vi "SetTrigger.vi"(8 "error in (no error)":errorcluster, 10 "Settings.Trigger":T1, 11 "PCO in":refnum<class "PCO_Camera.lvclass">) -> (0 "error out":errorcluster, 2 "Settings.Trigger  out":T1, 3 "PCO out":refnum<class "PCO_Camera.lvclass">)   [LabVIEW 2020, in "PCO_Camera.lvclass"]
uses:
  PCO_Camera.lvclass
  OnOffTypeDef.ctl
  PCO_Camera.lvclass/PCO_Camera.ctl
  Camera.lvclass
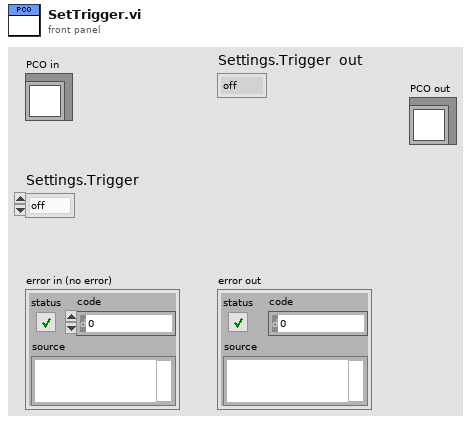
[diagram p1: front panel]
types:
  T1 = typedef "OnOffTypeDef.ctl" = enum16{"off", "on"}
  T2 = enum16{"sequence", "sequence non blocking", "ring buffer", "fifo", "sequence_dpcore", "sequence_non_blocking_dpcore", "ring_buffer_dpcore", "fifo_dpcore", "tif", "multitif", "pcoraw", "b16", "dicom", "multidicom"}
  T3 = enum16{"auto sequence", "software trigger", "external exposure start", "external exposure control"}
  T4 = typedef "Camera.lvclass/binning.ctl" = cluster{"vert":u16, "horz":u16}
  T5 = cluster{"exposure_time_s":dbl, "delay_time_s":dbl, "roi":cluster{"x0":u64, "y0":u64, "x1":u64, "y1":u64}, "timestamp_mode":u16, "pixelrate":u32, "trigger_mode":u16, "acquire_mode":u16, "metadata_mode":u16, "noisefilter_mode":u16, "binning":T4}
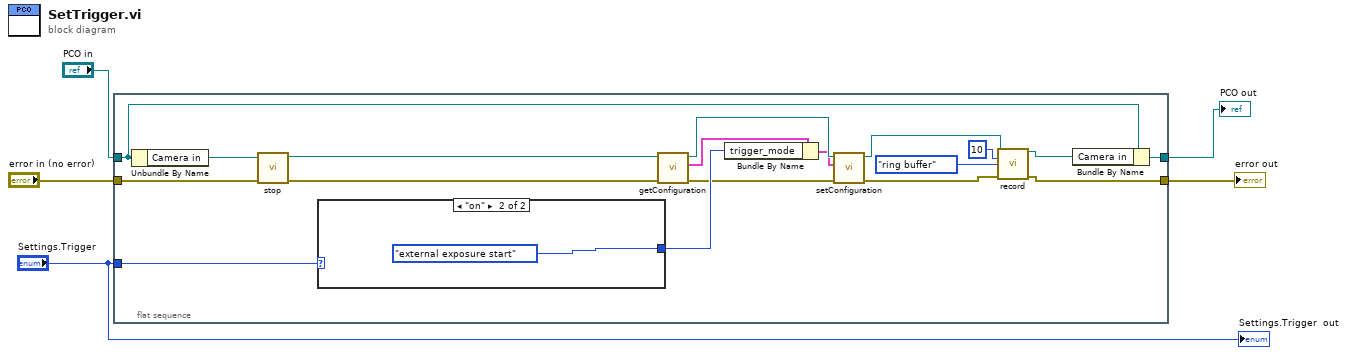
[diagram p0: block diagram]
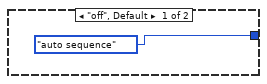
[diagram p2: hidden frame]
diagram:
  n1 = flat-sequence {
    tunnel: "error in (no error)" -> [w14]
    tunnel: "Settings.Trigger" -> [w20]
    tunnel: "PCO in" -> [w18]
    tunnel: [w9] -> w2
    tunnel: [w6] -> w1
    frame #0 {
      n2 = Unbundle By Name(w18) -> ("Camera in"=w16:refnum<class "Camera.lvclass">)
      n3 = call-dynamic "stop.vi"("error in (no error)"=w14, "Camera in"=w16) -> ("error out"=w13:errorcluster, "Camera out"=w15:refnum<class "Camera.lvclass">)  [unwired: 8 in]
      n4 = case shown="\"on\"" w20 {
        tunnel: [T3."auto sequence" ("TriggerMode") T3."external exposure start" ("TriggerMode")] -> w21
        frame "off", Default {
        }
        frame "on" {
        }
      }
      n5 = call-dynamic "getConfiguration.vi"("error in (no error)"=w13, "Camera in"=w15) -> ("error out"=w17:errorcluster, "configuration"=w22:T5, "Camera out"=w23:refnum<class "Camera.lvclass">)  [unwired: 7 in]
      n6 = Bundle By Name(cluster=w22, "trigger_mode"=w21) -> (w19:T5)
      n7 = call-dynamic "setConfiguration.vi"("error in (no error)"=w17, "configuration"=w19, "Camera in"=w23) -> ("error out"=w8:errorcluster, "Camera out"=w10:refnum<class "Camera.lvclass">)  [unwired: 7 in]
      n8 = call-dynamic "record.vi"("Camera in"=w10, "num_images"=u32 10, "record_mode"=T2."ring buffer", "error in (no error)"=w8) -> ("Camera out"=w7:refnum<class "Camera.lvclass">, "error out"=w9:errorcluster)  [unwired: 10 in]
      n9 = Bundle By Name(cluster=w18, "Camera in"=w7) -> (w6:refnum<class "PCO_Camera.lvclass">)
    }
  }
  "Settings.Trigger  out" <- "Settings.Trigger"
  "error out" <- w2
  "PCO out" <- w1
